vi "CRYTS New Insert.vi"() -> ()   [LabVIEW 2013]
uses:
  CRYSystem/Typedef Control/CRYStart Cluster.ctl
  CRYSystem/Typedef Control/CRYStep.ctl
  CRYSystem/Typedef Control/CRYTS.ctl
  CRYProject Editor Global.vi
  CRYSystem/Misc/SubVI/CRYMisc vis settings global.vi
  CRYMainGlobal.vi
panel:
  in  "TS":T1 {"Steps"."Repeat State Array"."Start" format="%#_5g"; "Steps"."Y dB ref" format="%.1f"; "Steps"."Y data" items=["dB", "Lin"]; "Steps"."Start" format="%#_5g"}
  in  "Step":T2 {"Repeat State Array"."Start" format="%#_5g"; "Y dB ref" format="%.1f"; "Y data" items=["dB", "Lin"]; "Start" format="%#_5g"}
  in  "Sequence Configure":T3
  # "Insert New Task Sequence."
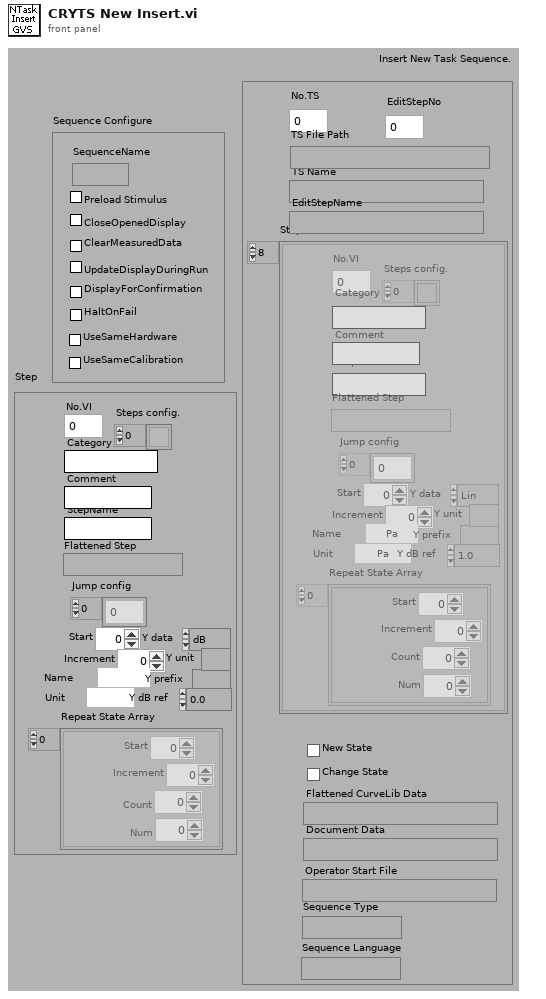
[diagram p1: front panel]
types:
  T1 = typedef "CRYTS.ctl" = cluster{"No.TS":u16, "TS File Path":path, "TS Name":string, "EditStepName":string, "Steps":T2[], "New State":bool, "Change State":bool, "Flattened CurveLib Data":string, "Document Data":string, "EditStepNo":u16, "Operator Start File":string, "Sequence Type":string, "Sequence Language":string}
  T2 = typedef "CRYStep.ctl" = cluster{"No.VI":i32, "Category":string, "StepName":string, "Seq setup flattened":string, "Comment":string, "Steps config.":bool[], "Jump config":i32[], "Start":dbl, "Increment":dbl, "Name":string, "Unit":string, "Y data":u16, "Y prefix":string, "Y dB ref":dbl, "Y unit":string, "Repeat State Array":cluster{"Start":dbl, "Increment":dbl, "Count":i32, "Num":i32}[]}
  T3 = typedef "CRYStart Cluster.ctl" = cluster{"SequenceName":string, "Preload Stimulus":bool, "CloseOpenedDisplay":bool, "ClearMeasuredData":bool, "UpdateDisplayDuringRun":bool, "DisplayForConfirmation":bool, "HaltOnFail":bool, "UseSameHardware":bool, "UseSameCalibration":bool}
  T4 = enum16{"New", "Open", "Close", "Close Data View Window Only", "Change", "Save", "Save for close"}
  T5 = typedef "CRYHardware.ctl" = cluster{"Name":string, "Analog I/O":u16, "Digital I/O":u16, "Channels":u8, "Dig Dev ID":u8, "N ports":u8, "Interface":u32, "Dig I/O Ports":cluster{"port #":i16, "width":i16, "direction":i32}[], "Interf settings":cluster{"Type":u16, "COM Port":u8, "Baud rate":u32, "Data bits":u32, "Parity":u16, "Stop bits":u16, "Flow control":u16, "Dev ID IEEE":u8}[], "N interfs":i32, "udev SNs":i16[], "udev enable":bool, "Channel Array":T6[], "Cal sequence":string, "SelectedIn":u16, "SelectedOut":u16, "SelectedTab":u16, "State":bool, "Help":string, "Advanced":bool, "In Audio Driver":u16, "Out Audio Driver":u16}
  T6 = typedef "CRYHardware Channel Info.ctl" = cluster{"ID":i32, "Name":string, "Digital":bool, "Input":bool, "Device Name":string, "Hardware Ch ID":u8, "Vmax (V)":dbl, "Latency (samples)":dbl, "Sampling Rate (Hz)":u32, "Bit Depth":u32, "Anti-aliasing Factor (%fs)":sgl, "DAQmx Channel":tag, "term config":i32, "Coupling":i32, "IEPE en":bool, "ASIOChannel Name":string, "Audio Driver":u16, "ASIOChannel Index":u8}
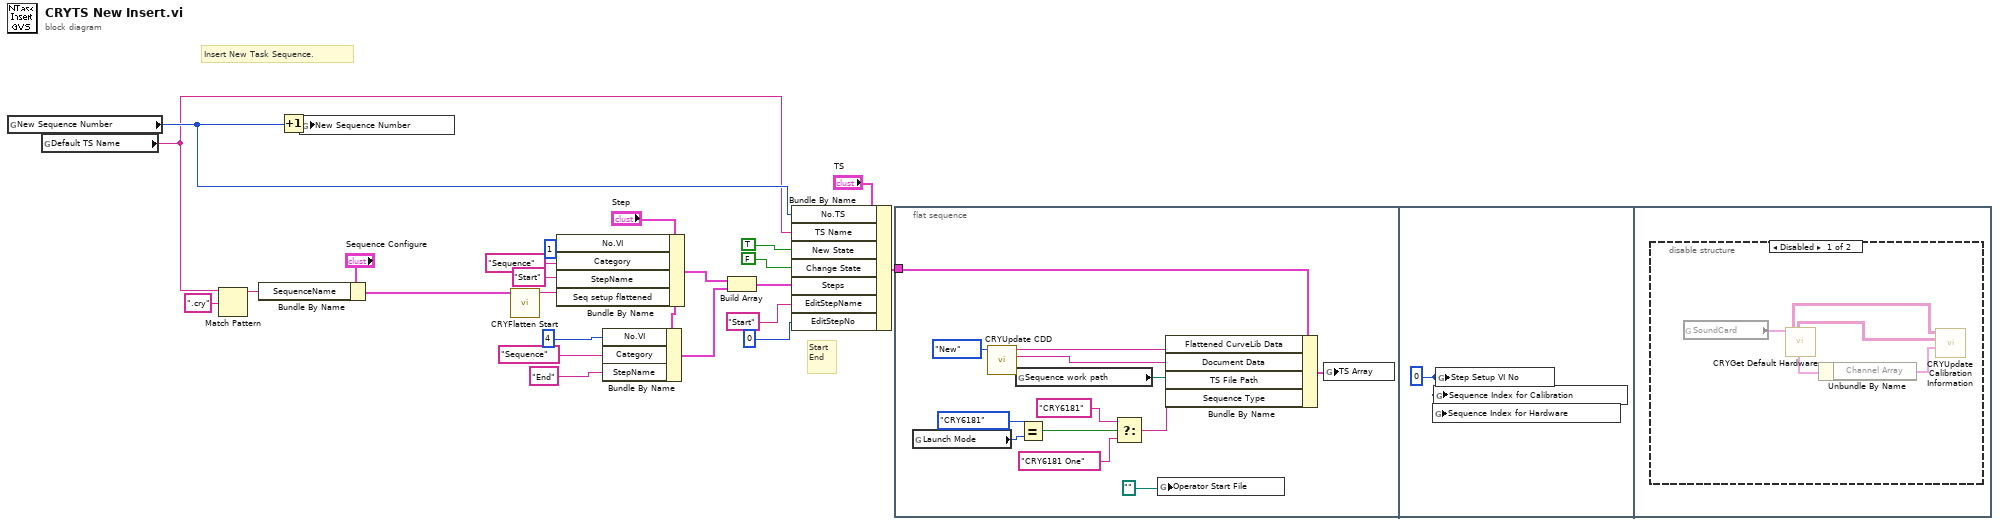
[diagram p0: block diagram]
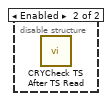
[diagram p2: hidden frame]
diagram:
  # "Start\nEnd"
  # "Insert New Task Sequence."
  n1 = global read "CRYProject Editor Global.vi" "New Sequence Number"() -> (w20:u16)
  n2 = global read "CRYProject Editor Global.vi" "Default TS Name"() -> (w7:string)
  n3 = Match Pattern(string=w7, regular expression=".cry") -> (before substring=w6:string)  [unwired: 1 in, 3 out]
  n4 = Bundle By Name(cluster="Sequence Configure", "SequenceName"=w6) -> (w14:T3)
  n5 = Increment(x=w20) -> (x+1=w21:u16)
  n6 = global write "CRYProject Editor Global.vi" "New Sequence Number"(w21) -> ()
  n7 = call "CRYFlatten Start.vi"("Start"=w14) -> ("Start flattened"=w13:string)  [unwired: 10 in]
  n8 = Bundle By Name(cluster="Step", "No.VI"=1, "Category"="Sequence", "StepName"="Start" ("Category"), "Seq setup flattened"=w13) -> (w3:T2)
  n9 = Bundle By Name(cluster="Step", "No.VI"=4, "Category"="Sequence", "StepName"="End" ("Category")) -> (w1:T2)
  n10 = Build Array(w3, w1) -> (w22:T2[])
  n11 = Bundle By Name(cluster="TS", "No.TS"=w20, "TS Name"=w7, "New State"=TRUE, "Change State"=FALSE, "Steps"=w22, "EditStepName"="Start", "EditStepNo"=u16 0) -> (w18:T1)
  n12 = flat-sequence {
    tunnel: w18 -> [w33]
    frame #0 {
      n13 = global read "CRYMainGlobal.vi" "Launch Mode"() -> (w27:enum32{"CRY6181", "CRY6181 One"})
      n14 = call "CRYUpdate CDD.vi"("Signal"=T4."New") -> ("Document Data Out"=w36:string, "Flatten Data Out"=w35:string)  [unwired: 2 in, 7 out]
      n15 = global read "CRYMainGlobal.vi" "Sequence work path"() -> (w32:path)
      n16 = Equal?(x=enum32{"CRY6181", "CRY6181 One"}."CRY6181", y=w27) -> (x = y?=w26:bool)
      n17 = Select(t="CRY6181" ("Section"), s=w26, f="CRY6181 One" ("Section")) -> (s? t:f=w28:string)
      n18 = global write "CRYMisc vis settings global.vi" "Operator Start File"(path "") -> ()
      n19 = Bundle By Name(cluster=w33, "Flattened CurveLib Data"=w35, "Document Data"=w36, "TS File Path"=w32, "Sequence Type"=w28) -> (w34:T1)
      n20 = global write "CRYProject Editor Global.vi" "TS Array"(w34) -> ()
    }
    frame #1 {
      w38 = 0 ("Docked  VI No")
      n21 = global write "CRYProject Editor Global.vi" "Sequence Index for Hardware"(w38) -> ()
      n22 = global write "CRYProject Editor Global.vi" "Sequence Index for Calibration"(w38) -> ()
      n23 = global write "CRYProject Editor Global.vi" "Step Setup VI No"(w38) -> ()
    }
    frame #2 {
      n24 = disable-structure shown="Disabled" {
        frame Disabled {
          n25 = global read "CRYProject Editor Global.vi" "SoundCard"() -> (w43:T5)
          n26 = call "CRYGet Default Hardware.vi"("Hardware Cluster In"=w43) -> ("I_Name Out"=w40:string[][], "O_Name Out"=w39:string[][], "Hardware Cluster Out"=w42:T5)  [unwired: 16 out]
          n27 = Unbundle By Name(w42) -> ("Channel Array"=w41:T6[])
          n28 = call "CRYUpdate Calibration Information.vi"("Hardware Channel Array"=w41, "O_Name In"=w39, "I_Name In"=w40) -> ()  [unwired: 1 in, 8 out]
        }
        frame Enabled {
          n29 = call "CRYCheck TS After TS Read.vi"() -> ()  [unwired: 1 out]
        }
      }
    }
  }
